vi "Get Trigger ID.vi"(11 "FRTS Process in":refnum<class "FRTS Process.lvclass">) -> (2 "Trigger ID":u8, 3 "FRTS Process out":refnum<class "FRTS Process.lvclass">)   [LabVIEW 2019, in "TimingDRV Engine.lvlib" / "FRTS Process.lvclass"]
uses:
  FRTS Process.lvclass
  FRTS Process.lvclass/FRTS Process.ctl
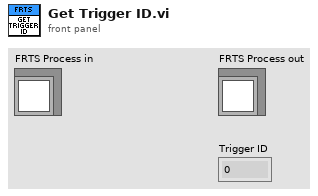
[diagram p1: front panel]
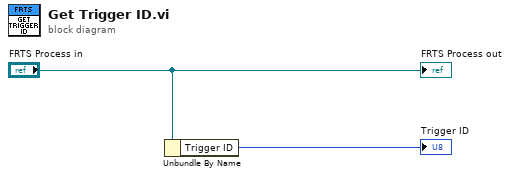
[diagram p0: block diagram]
diagram:
  n1 = Unbundle By Name("FRTS Process in") -> ("Trigger ID"=→"Trigger ID":u8)
  "FRTS Process out" <- "FRTS Process in"
